vi "FisherPaykel Set Direction and Runtime.vi"(4 "GEA Inputs":T1={"Source"=228, "Destination"=35} {"Destination" format="%.0x"; "Source" format="%.0x"}, 5 "Use GEA Inverter Output":bool, 6 "Main Command":T4=">GS", 7 "Debug":bool, 8 "error in (no error)":errorcluster, 9 "GEA2 Reference In":refnum<k24>, 10 "Spin Profile":T2={"Target Speed (RPM)"=23, "Acceleration Rate - (10 Slowest/1000 Fastest)"=20, "Running Time (s)"=20, "Direction (CW or CCW)"=""} {"Running Time (s)" step=1; "Acceleration Rate - (10 Slowest/1000 Fastest)" min=10 max=1000 step=1; "Target Speed (RPM)" min=23 max=1600 step=1}, 11 "VISA Refnum in":refnum<visa-resource-name>="COM3") -> (0 "error out":errorcluster, 1 "GEA2 Reference Out":refnum<k24>, 2 "Command (Debug)":string, 3 "VISA Refnum out":refnum<visa-resource-name>="COM3")   [LabVIEW 2016]
uses:
  Type Definitions/Fisher Paykel Main Command.ctl
  Type Definitions/Fisher Paykel Motor Profile.ctl
  Type Definitions/FisherPaykel Direction CMD.ctl
  Trunk/Utility/LabVIEW GEA2 Toolkit v1.0.0.0/type defs/Source_Destination.ctl
  C:/Technology Lab/NI-2010/Trunk/Utility/LabVIEW GEA2 Toolkit v1.0.0.0/Appliance.NET/GeaCommunication.dll
  Trunk/Utility/LabVIEW GEA2 Toolkit v1.0.0.0/Appliance.NET/GeaCommunication.dll
  Trunk/Utility/LabVIEW GEA2 Toolkit v1.0.0.0/type defs/ERD Write Data In.ctl
  Trunk/Utility/LabVIEW GEA2 Toolkit v1.0.0.0/type defs/Data Type.ctl
  Trunk/Utility/LabVIEW GEA2 Toolkit v1.0.0.0/library/GEA2_Toolkit.lvlib
panel:
  # "Spin Profile Parameters"
  # "Spin Start Parameters"
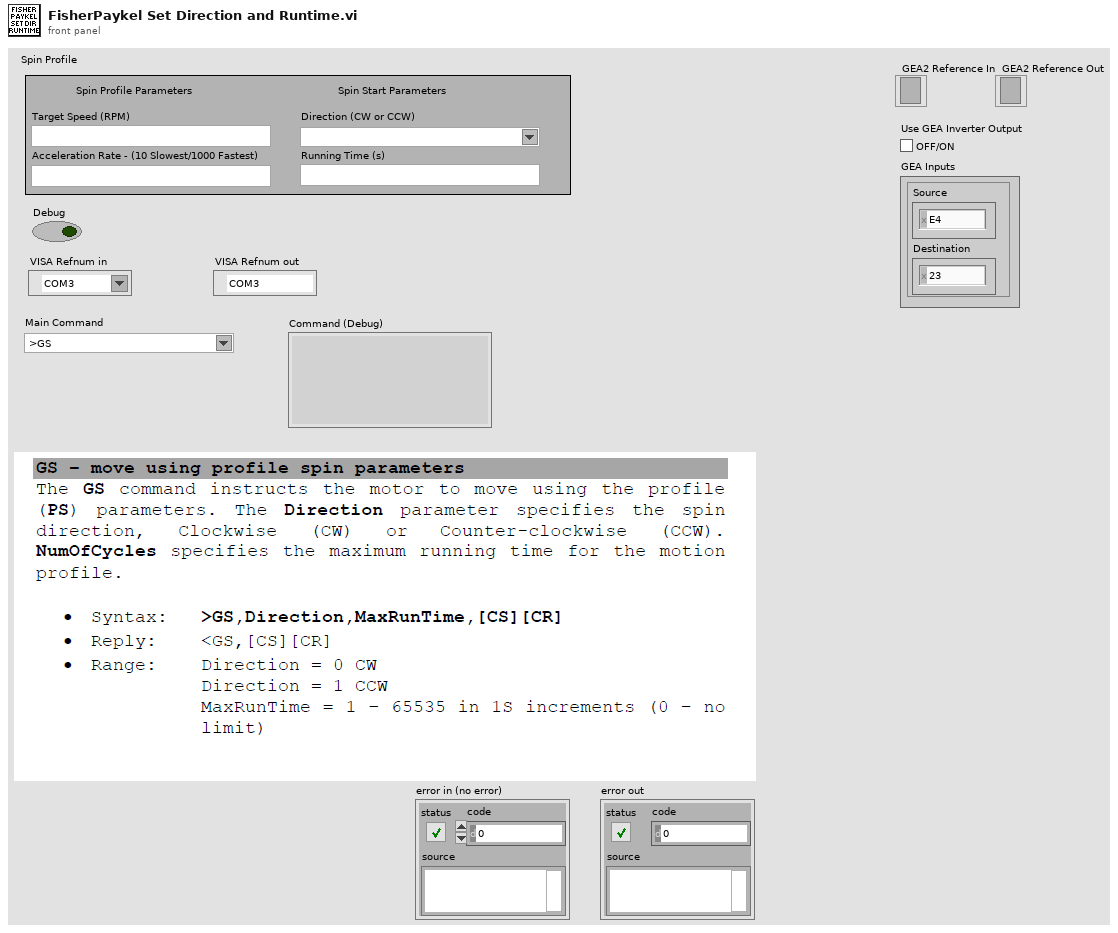
[diagram p1: front panel]
types:
  T1 = typedef "GEA2_Toolkit.lvlib/Source_Destination.ctl" = cluster{"Source":u8, "Destination":u8}
  T2 = typedef "Fisher Paykel Motor Profile.ctl" = cluster{"Target Speed (RPM)":u16, "Acceleration Rate - (10 Slowest/1000 Fastest)":u16, "Running Time (s)":u16, "Direction (CW or CCW)":T3}
  T3 = typedef "FisherPaykel Direction CMD.ctl" = string
  T4 = typedef "Fisher Paykel Main Command.ctl" = string
  T5 = typedef "GEA2_Toolkit.lvlib/ERD Write Data In.ctl" = cluster{"ERD Number":u16, "Data Type":T6, "Data":string}
  T6 = typedef "GEA2_Toolkit.lvlib/Data Type.ctl" = enum16{"string", "boolean", "uint8_t", "uint16_t", "uint32_t", "uint64_t"}
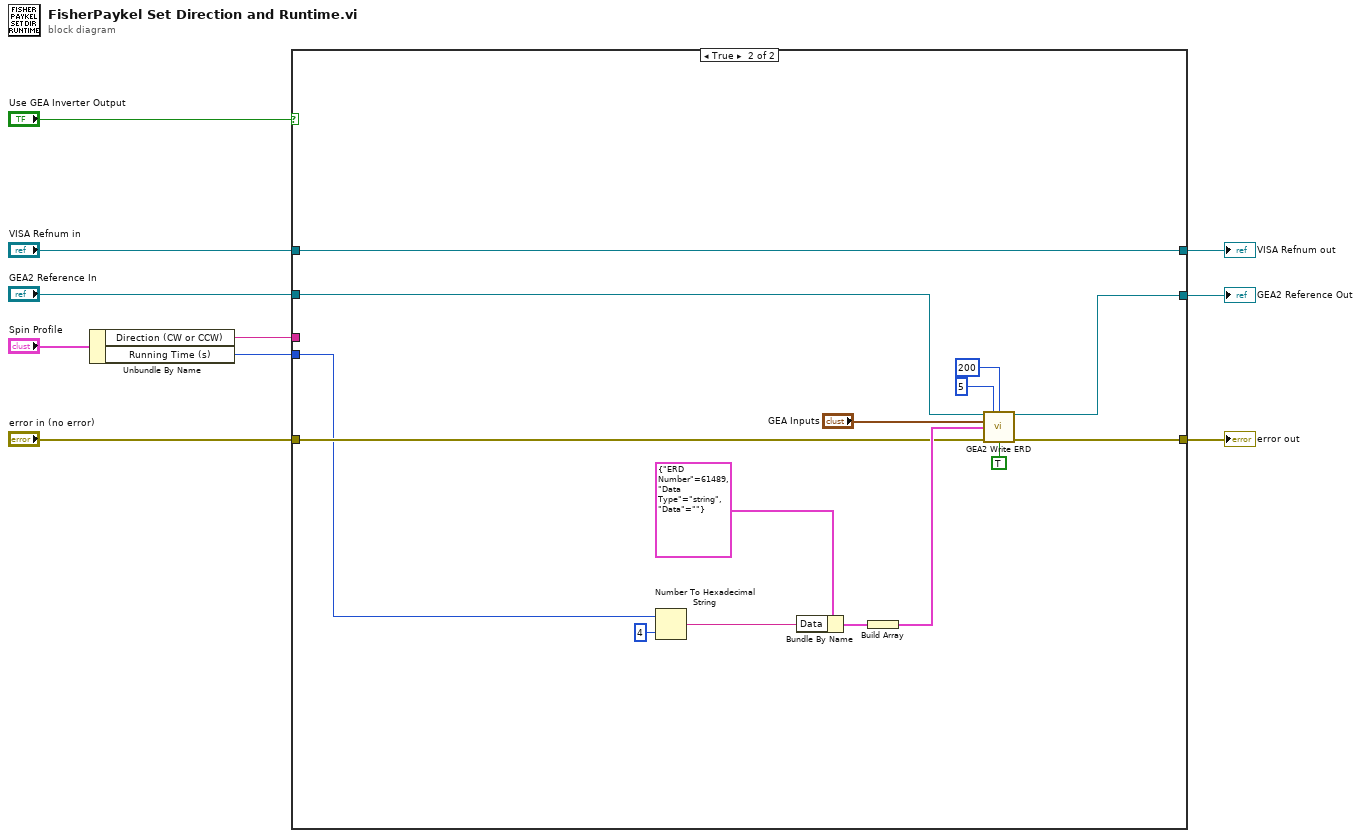
[diagram p0: block diagram]
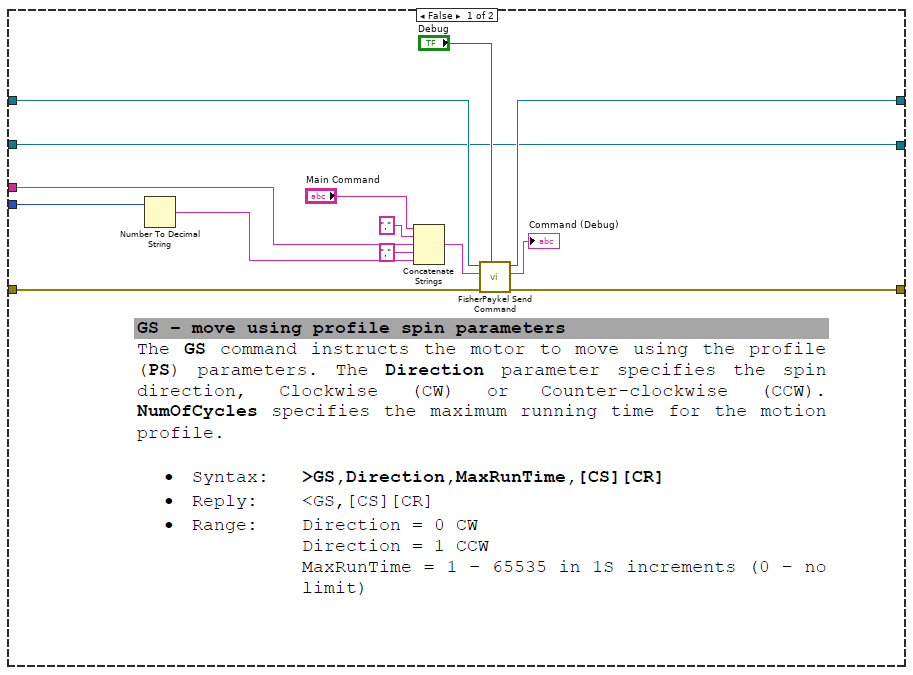
[diagram p2: hidden frame]
diagram:
  n1 = Unbundle By Name("Spin Profile") -> ("Direction (CW or CCW)"=w5:T3, "Running Time (s)"=w4:u16)
  n2 = case shown="True" "Use GEA Inverter Output" {
    tunnel: "VISA Refnum in" -> [w21 w39]
    tunnel: "error in (no error)" -> [w20 w31]
    tunnel: [w18 w39] -> w8
    tunnel: [w17 w30] -> w7
    tunnel: w5 -> [w14 _]
    tunnel: w4 -> [w13 w27]
    tunnel: [w11 w29] -> w2
    tunnel: "GEA2 Reference In" -> [w11 w28]
    frame False {
      n3 = Number To Decimal String(number=w13) -> (decimal integer string=w12:string)  [unwired: 1 in]
      n4 = Concatenate Strings("Main Command", ",", w14, "," ("string"), w12) -> (w19:string)
      n5 = call "FisherPaykel Send Command.vi"("Debug"="Debug", "error in (no error)"=w20, "Send Command"=w19, "VISA Refnum in"=w21) -> ("error out"=w17:errorcluster, "Command (Debug)"=→"Command (Debug)":string, "VISA Refnum out"=w18:refnum<visa-resource-name>)  [unwired: 5 in]
    }
    frame True {
      n6 = Number To Hexadecimal String(1:i16 4 ("width (-)"), 2:w27) -> (0:w25:string)
      n7 = Bundle By Name(cluster=T5 {"ERD Number"=61489, "Data Type"=enum."string", "Data"=""} ("ERD Write Data In"), "Data"=w25) -> (w38:T5)
      n8 = Build Array(w38) -> (w36:T5[])
      n9 = call "GEA2 Write ERD.vi"("GEA2 Reference In"=w28, "Retry Count"=5, "Read Timeout (ms)"=u32 200, "GEA Inputs"="GEA Inputs", "Write ERD List"=w36, "Error In"=w31, "Verify ERD Response?"=TRUE) -> ("GEA2 Reference Out"=w29:refnum<k24>, "Error Out"=w30:errorcluster)  [unwired: 6 in, 1 out]
    }
  }
  "error out" <- w7
  "VISA Refnum out" <- w8
  "GEA2 Reference Out" <- w2
